vi "Client Panel.vi"() -> ()   [LabVIEW 2017]
uses:
  <vilib>/Rock Robotics/Network Tables/NT Read Numeric Array.vi
  <vilib>/Rock Robotics/Network Tables/NT Read String Array.vi
panel:
  in  "String 2":string
  in  "Numeric":dbl
  in  "Boolean 3":bool
  in  "Dbl 2":dbl
  in  "Boolean 2":bool
  in  "ms between reads":u32=100
  out "Boolean":bool
  out "String":string
  out "Dbl":dbl
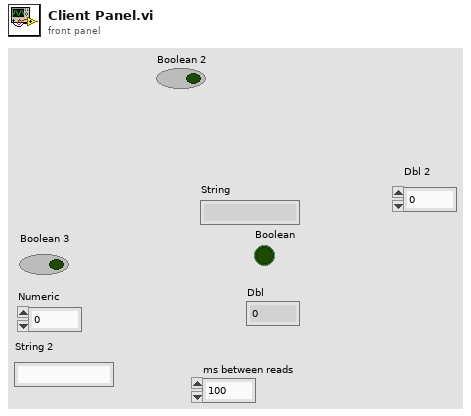
[diagram p1: front panel]
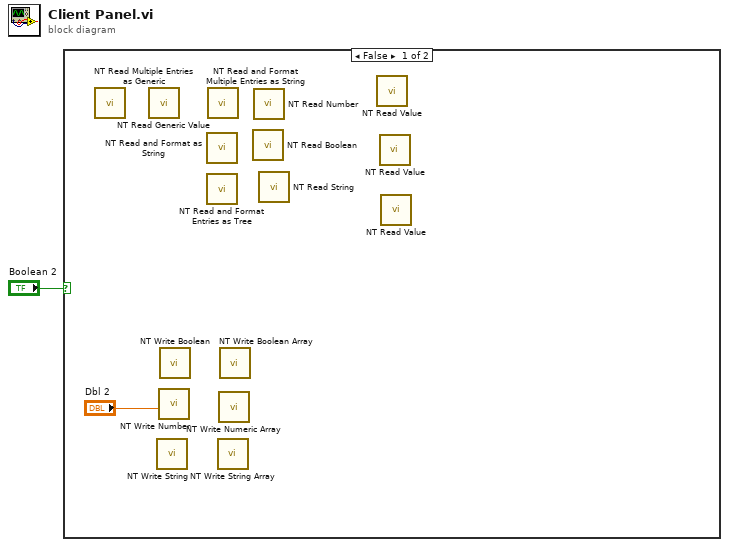
[diagram p0: block diagram]
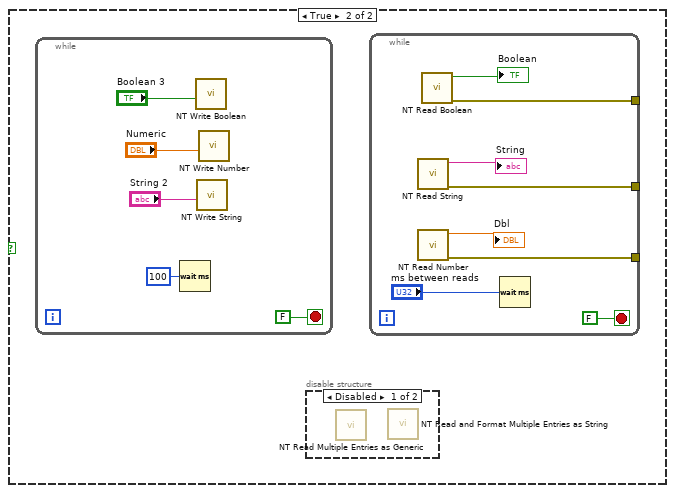
[diagram p2: hidden frame]
diagram:
  n1 = case shown="False" "Boolean 2" {
    frame False {
      n2 = call <vilib>:"NT Read Multiple Entries as Generic.vi"() -> ()  [unwired: 9 in, 3 out]
      n3 = call <vilib>:"NT Read Generic Value.vi"() -> ()  [unwired: 10 in, 2 out]
      n4 = call <vilib>:"NT Write String.vi"() -> ()  [unwired: 11 in, 1 out]
      n5 = call <vilib>:"NT Write Number.vi"("Numeric"="Dbl 2") -> ()  [unwired: 10 in, 1 out]
      n6 = call <vilib>:"NT Write Boolean.vi"() -> ()  [unwired: 11 in, 1 out]
      n7 = call <vilib>:"NT Read and Format as String.vi"() -> ()  [unwired: 11 in, 1 out]
      n8 = call <vilib>:"NT Read and Format Entries as Tree.vi"() -> ()  [unwired: 10 in, 2 out]
      n9 = call <vilib>:"NT Read and Format Multiple Entries as String.vi"() -> ()  [unwired: 10 in, 2 out]
      n10 = call <vilib>:"NT Write String Array.vi"() -> ()  [unwired: 11 in, 1 out]
      n11 = call <vilib>:"NT Write Numeric Array.vi"() -> ()  [unwired: 11 in, 1 out]
      n12 = call <vilib>:"NT Write Boolean Array.vi"() -> ()  [unwired: 11 in, 1 out]
      n13 = call <vilib>:"NT Read Boolean.vi"() -> ()  [unwired: 10 in, 2 out]
      n14 = call <vilib>:"NT Read Number.vi"() -> ()  [unwired: 10 in, 2 out]
      n15 = call <vilib>:"NT Read String.vi"() -> ()  [unwired: 10 in, 2 out]
      n16 = call-poly <vilib>:"NT Read Value.vi"() -> ()  [unwired: 10 in, 2 out]
      n17 = call-poly <vilib>:"NT Read Value.vi"() -> ()  [unwired: 10 in, 2 out]
      n18 = call-poly <vilib>:"NT Read Value.vi"() -> ()  [unwired: 10 in, 2 out]
    }
    frame True {
      n19 = while {
        stop <- FALSE stop-if-true
        n20 = Wait (ms)(milliseconds to wait=u32 100) -> ()  [unwired: 1 out]
        n21 = call <vilib>:"NT Write Boolean.vi"("Boolean"="Boolean 3") -> ()  [unwired: 10 in, 1 out]
        n22 = call <vilib>:"NT Write String.vi"("String"="String 2") -> ()  [unwired: 10 in, 1 out]
        n23 = call <vilib>:"NT Write Number.vi"("Numeric"="Numeric") -> ()  [unwired: 10 in, 1 out]
      }
      n24 = disable-structure shown="Disabled" {
        frame Disabled {
          n25 = call <vilib>:"NT Read Multiple Entries as Generic.vi"() -> ()  [unwired: 9 in, 3 out]
          n26 = call <vilib>:"NT Read and Format Multiple Entries as String.vi"() -> ()  [unwired: 10 in, 2 out]
        }
        frame Enabled {
        }
      }
      n27 = while {
        tunnel: [w10] -> _
        tunnel: [w9] -> _
        tunnel: [w8] -> _
        stop <- FALSE stop-if-true
        n28 = call <vilib>:"NT Read String.vi"() -> ("error out"=w9:errorcluster, "String"=→"String":string)  [unwired: 10 in]
        n29 = call <vilib>:"NT Read Number.vi"() -> ("error out"=w8:errorcluster, "Numeric"=→"Dbl":dbl)  [unwired: 10 in]
        n30 = call <vilib>:"NT Read Boolean.vi"() -> ("error out"=w10:errorcluster, "Boolean"=→"Boolean":bool)  [unwired: 10 in]
        n31 = Wait (ms)(milliseconds to wait="ms between reads") -> ()  [unwired: 1 out]
      }
    }
  }
